vi "To Variant.vi"(0 "Obj in":refnum<class "Tone Cloud.lvclass">, 11 "error in (no error)":errorcluster) -> (4 "Obj out":refnum<class "Tone Cloud.lvclass">, 8 "Array":variant[](array[variant]), 15 "error out":errorcluster)   [LabVIEW 2020, in "Tone Cloud.lvclass"]
uses:
  Tone Cloud.lvclass
  Tone Cloud.lvclass/Tone Cloud.ctl
  Waveform/Waveform.lvclass
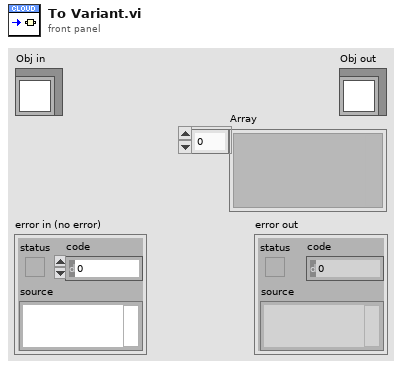
[diagram p1: front panel]
types:
  T1 = typedef "Tone Cloud.lvclass/Serialized.ctl" = cluster{"Fmin (Hz)":dbl, "Fmax (Hz)":dbl, "Spacing":T2, "Components/oct":dbl, "Level (dB)":string, "Level mode":T3, "Density":string, "Pip ramp (ms)":dbl, "Pip duration (ms)":dbl, "Pip rate (Hz)":dbl, "Seed":i32, "Tokens":i32, "Plot mask":bool}
  T2 = typedef "Tone Cloud.lvclass/Spacing.ctl" = enum16{"Linear", "Log"}
  T3 = typedef "Tone Cloud.lvclass/Level Mode.ctl" = enum16{"per component", "total rms"}
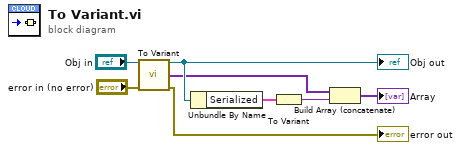
[diagram p0: block diagram]
diagram:
  n1 = call-parent "To Variant.vi"("Obj in"="Obj in", "error in (no error)"="error in (no error)") -> ("Obj out"=w3:refnum<class "Tone Cloud.lvclass">, "Array"=w2:variant[], "error out"=→"error out":errorcluster)  [unwired: 11 in]
  "Obj out" <- w3
  n2 = Unbundle By Name(w3) -> ("Serialized"=w4:T1)
  n3 = To Variant(anything=w4) -> (Variant=w5:variant)
  n4 = Build Array (concatenate)(w2, w5) -> (→"Array":variant[])
